vi "Car Wash.vi"() -> ()   [LabVIEW 2020]
uses:
  Controls/Car Wash Indicators.ctl
  Controls/Wash Options.ctl
  Controls/Car Wash References.ctl
  Controls/Wash Steps Selected-Update Display Message.ctl
  Controls/Timer Controls.ctl
  Support/Enqueue Message (Single).vi
  <vilib>/Utility/error.llb/Error Cluster From Error Code.vi
  <vilib>/ErrorRing/Error Ring.xnode
  Support/Message Queue.lvlib
panel:
  in  "Start":bool
  out "Elapsed Time":dbl format="%0.2f"
  in  "stop":bool
  out "Wash Entry":bool
  in  "Wash Options":T1
  in  "Car Position Slider":u8(slide) max=3 scale=0.0..4.0
  out "Car Wash Indicators":T2
  # "Entry Console"
  # "Car Wash Display"
  # "Car Position Simulation"
  # "Pre-Soak\nH-P Wash\nL-P Wax\nSpot Free Rinse"
  # "Underbody Wash\nBug Remover"
  # "Tire Shine\nAir Dry"
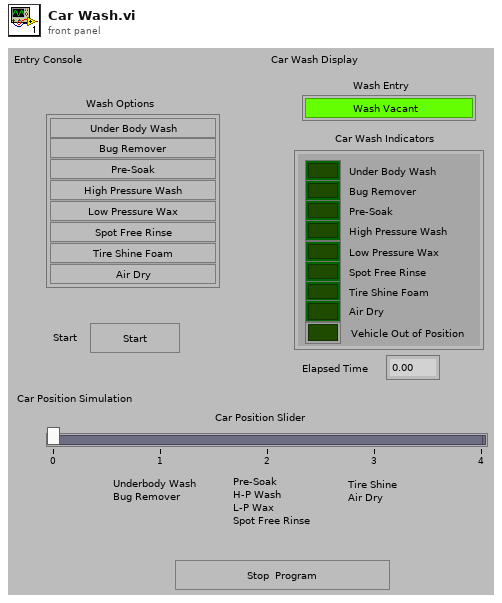
[diagram p1: front panel]
types:
  T1 = typedef "Wash Options.ctl" = cluster{"Underbody Wash":bool, "Bug Remover":bool, "Pre-Soak":bool, "High Pressure Wash":bool, "Low Pressure Wax":bool, "Spot Free Rinse":bool, "Tire Shine Foam":bool, "Air Dry":bool}
  T2 = typedef "Car Wash Indicators.ctl" = cluster{"Under Body Wash":bool, "Bug Remover":bool, "Pre-Soak":bool, "High Pressure Wash":bool, "Low Pressure Wax":bool, "Spot Free Rinse":bool, "Tire Shine Foam":bool, "Air Dry":bool, "Vehicle Out of Position":bool}
  T3 = typedef "Car Wash References.ctl" = cluster{"Car Wash Indicators Ref":refnum<vi>, "Wash Options Ref":refnum<vi>, "Car Position Slider Ref":refnum<vi>, "Elapsed Time Ref":refnum<vi>, "Wash Entry Ref":refnum<vi>, "Start Ref":refnum<vi>}
  T4 = typedef "Message Queue.lvlib/All Message Queues.ctl" = cluster{"UI":refnum<queue>}
  T5 = typedef "Wash Steps Selected-Update Display Message.ctl" = cluster{"Wash Steps Selected":cluster{"Wash Step":string, "Step Time":i32, "Station":string}[], "Update Display Message":string}
  T6 = enum8{"Enabled", "Disabled", "Disabled and Grayed Out"}
  T7 = typedef "Timer Controls.ctl" = enum16{"Reset", "Start", "Stop"}
  T8 = cluster{"Wash Step":string, "Step Time":i32, "Station":string}[]
  T9 = cluster{"Wash Step":string, "Step Time":i32, "Station":string}
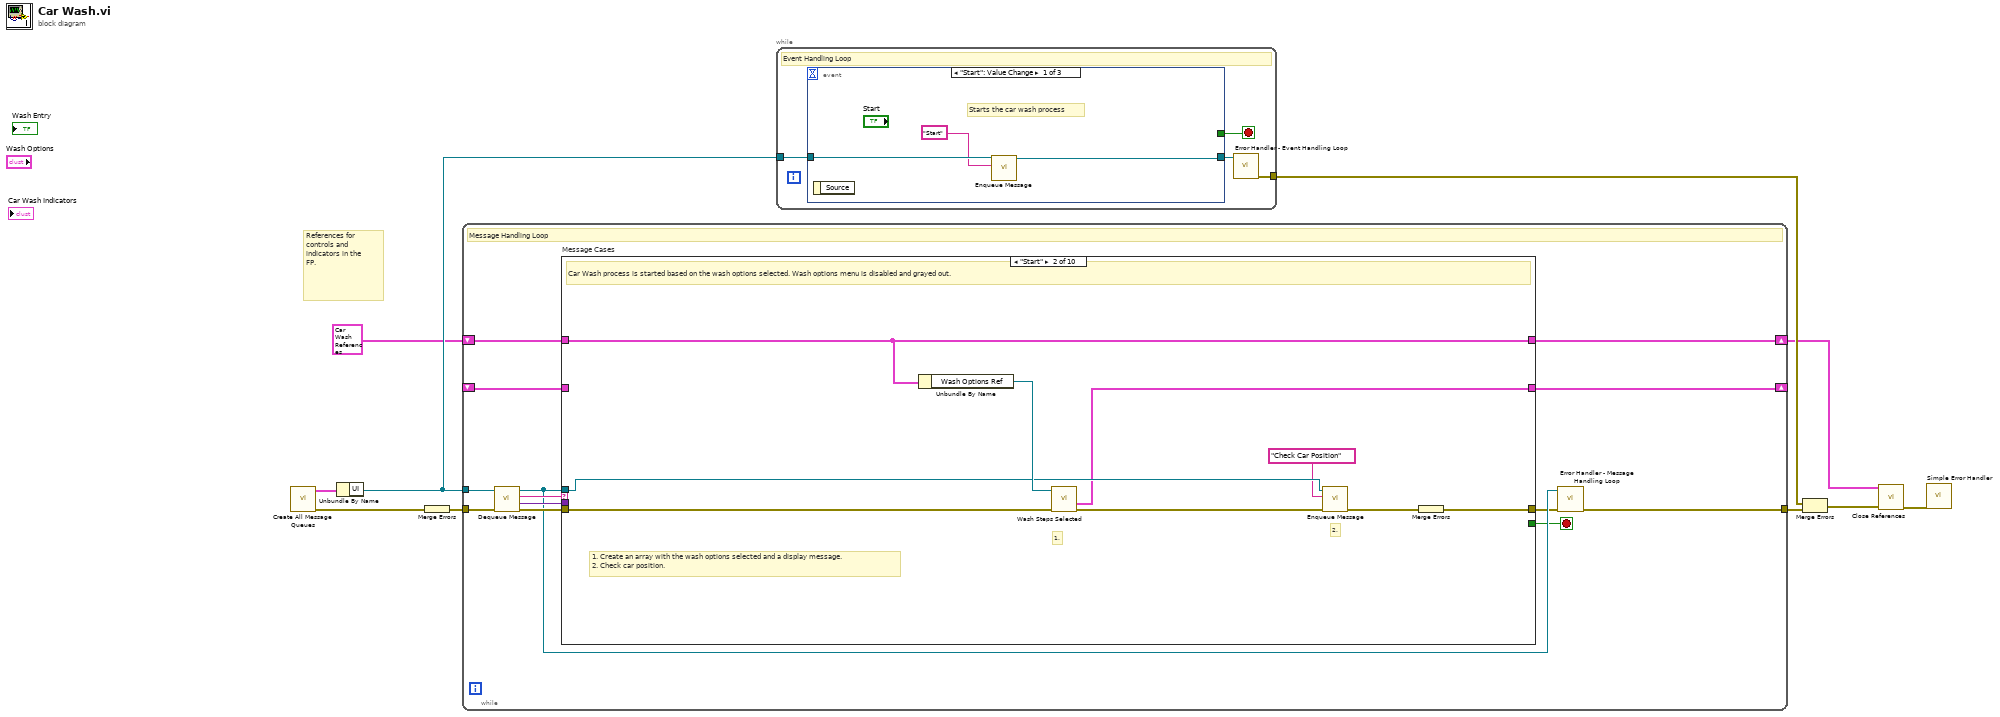
[diagram p0: block diagram]
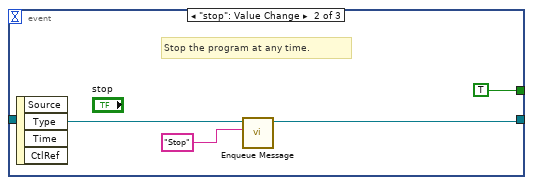
[diagram p2: hidden frame]
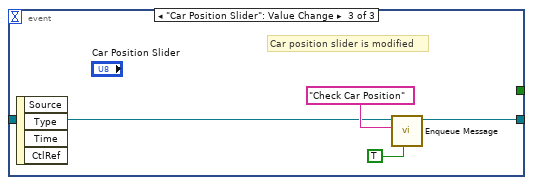
[diagram p3: hidden frame]
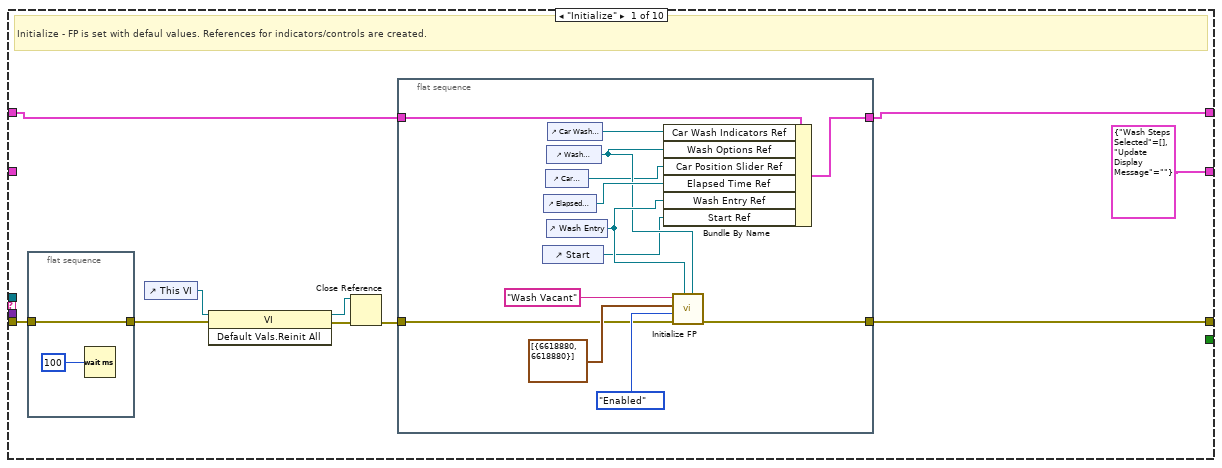
[diagram p4: hidden frame]
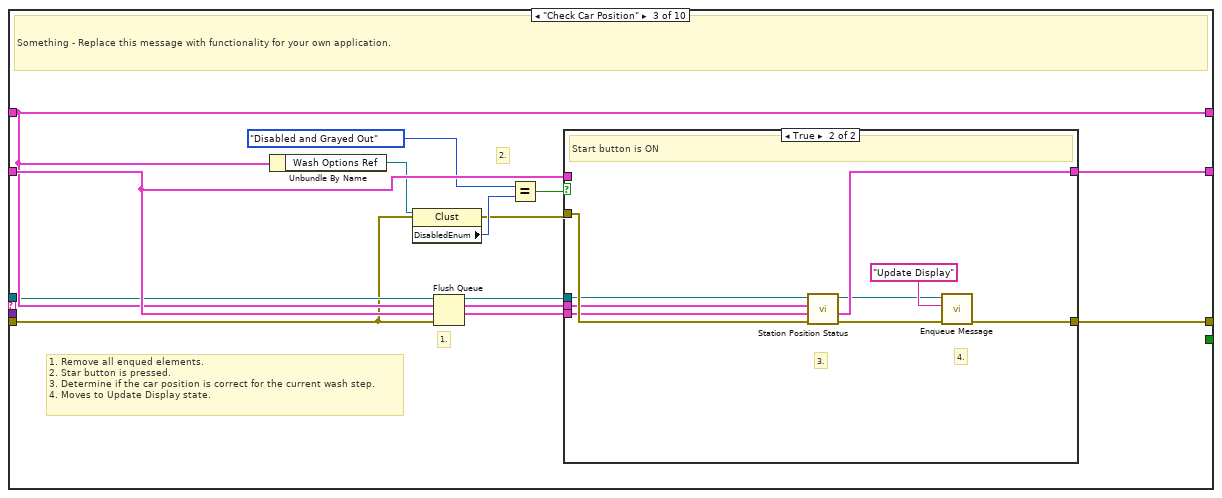
[diagram p5: hidden frame]
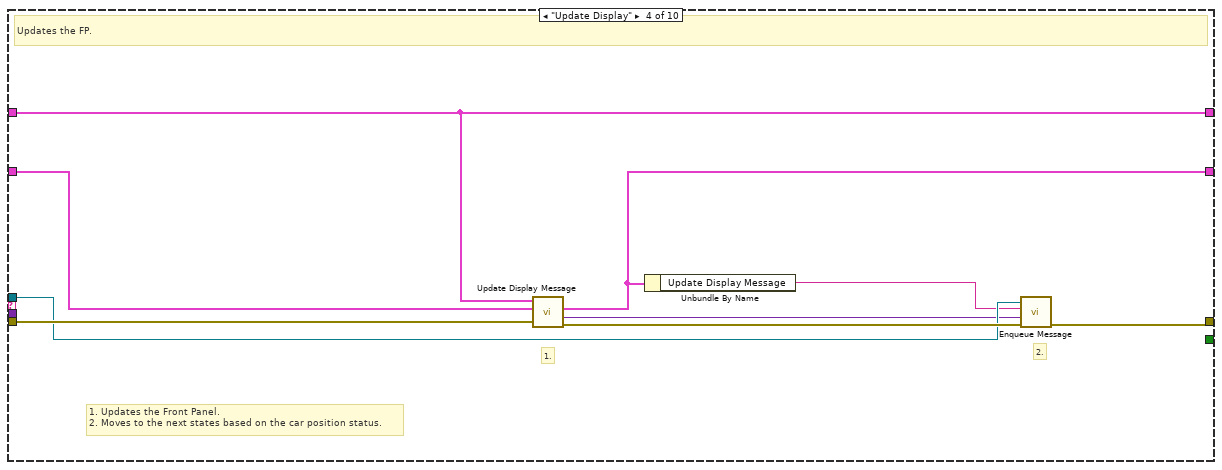
[diagram p7: hidden frame]
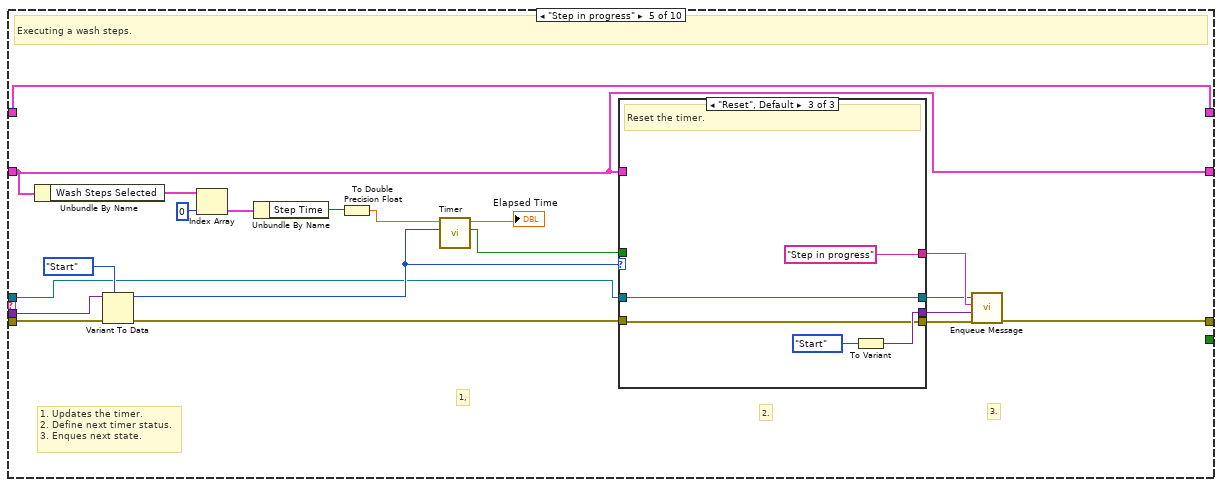
[diagram p8: hidden frame]
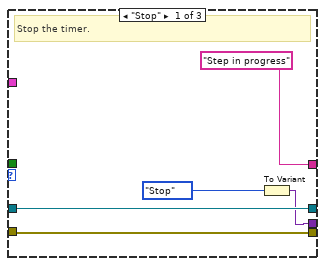
[diagram p9: hidden frame]
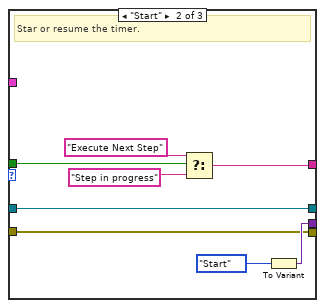
[diagram p10: hidden frame]
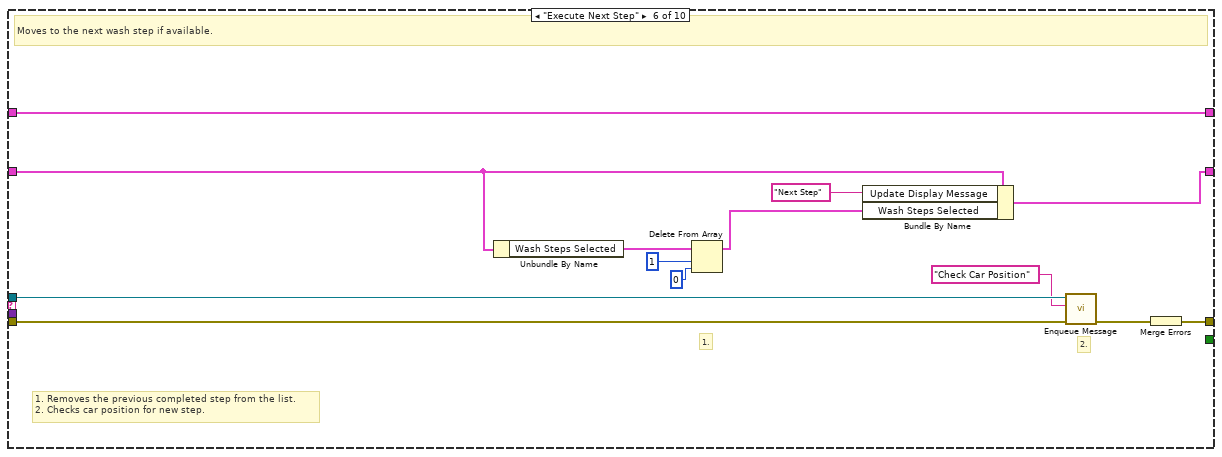
[diagram p11: hidden frame]
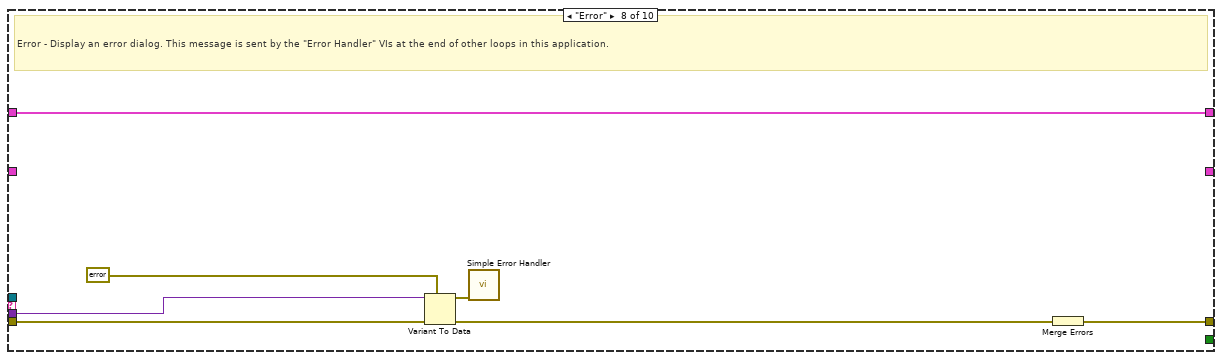
[diagram p13: hidden frame]
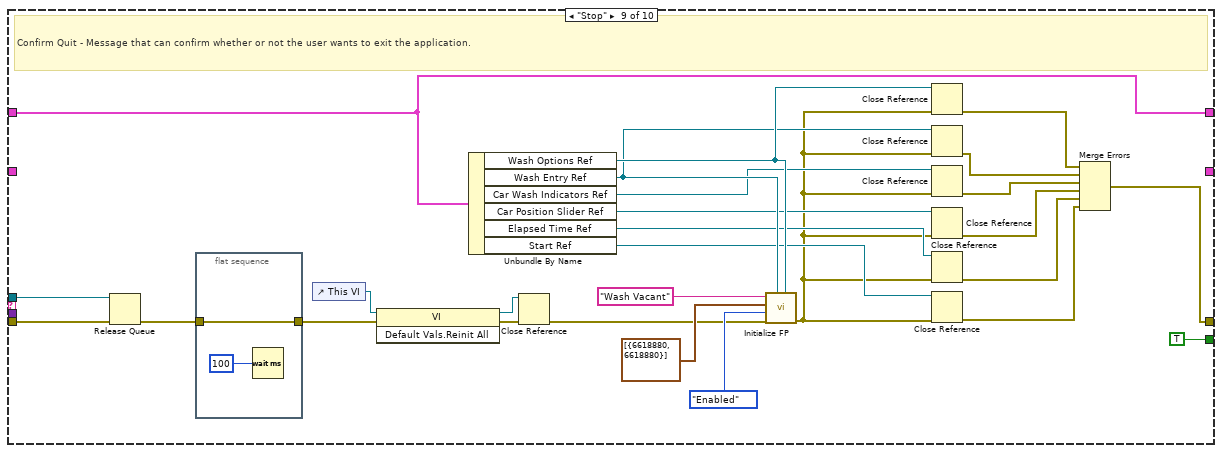
[diagram p14: hidden frame]
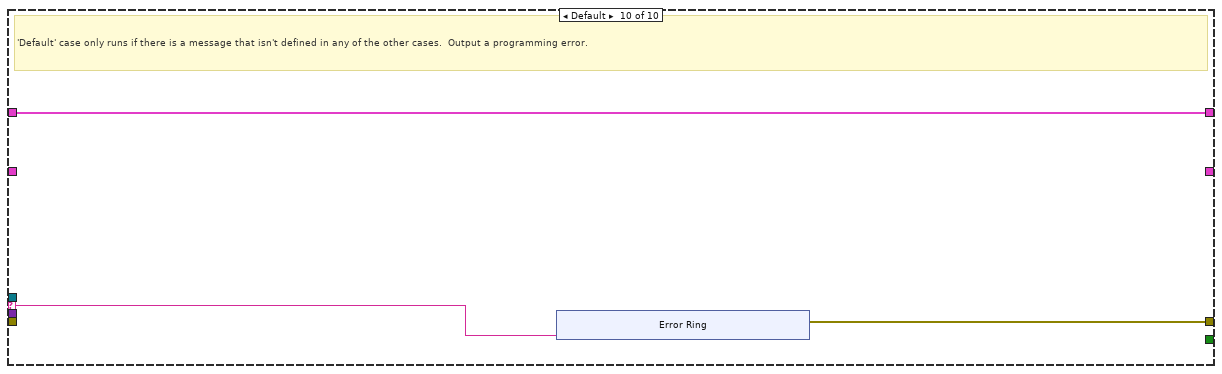
[diagram p15: hidden frame]
diagram:
  # "References for controls and indicators in the FP."
  n1 = call "Create All Message Queues.vi"() -> ("error out"=w10:errorcluster, "Message Queues out"=w9:T4)  [unwired: 10 in]
  n2 = Unbundle By Name(w9) -> ("UI"=w7:refnum<queue>)
  n3 = Merge Errors(w10) -> (w5:errorcluster)
  n4 = while {
    tunnel: w7 -> [w17]
    shift-right: [w22] -> w3
    shift-left: T3 {"Car Wash Indicators Ref"=refnum, "Wash Options Ref"=refnum, "Car Position Slider Ref"=refnum, "Elapsed Time Ref"=refnum, "Wash Entry Ref"=refnum, "Start Ref"=refnum} ("Data Cluster") -> [w23]
    tunnel: w5 -> [w21]
    tunnel: [w15] -> w8
    shift-right: [w12] -> _
    shift-left: _ -> [w11]
    stop <- w13 stop-if-true
    # "Message Handling Loop"
    n5 = call "Dequeue Message.vi"("error in (no error)"=w21, "Message Queue"=w17) -> ("error out"=w20:errorcluster, "Message Data"=w18:variant, "Message"=w19:string, "dup Message Queue"=w16:refnum<queue>)  [unwired: 6 in]
    n6 = case "Message Cases" shown="\"Start\"" w19 {
      selector: w19 -> [_ _ _ _ _ _ _ _ _ w179]
      tunnel: w16 -> [_ w52 w59 w84 w93 w136 _ _ w175 _]
      tunnel: w20 -> [w28 w55 w58 w88 w102 w128 w140 w149 w174 _]
      tunnel: [w29 w57 w69 w85 w94 w138 w140 w143 w151 w180] -> w14
      tunnel: w23 -> [w33 w56 w66 w87 w108 w139 w142 w148 w150 w181]
      tunnel: [w31 w56 w66 w87 w108 w139 w142 w148 w150 w181] -> w22
      tunnel: w18 -> [_ _ _ _ w103 _ _ w147 _ _]
      tunnel: [_ _ _ _ _ _ _ _ TRUE _] -> w13
      tunnel: [T5 {"Wash Steps Selected"=[], "Update Display Message"=""} ("Wash Steps Selected-Update Display Message") w50 w68 w81 w91 w127 w141 _ _ _] -> w12
      tunnel: w11 -> [_ _ w67 w82 w91 w131 w141 _ _ _]
      frame "Initialize" {
        # "Initialize - FP is set with defaul values. References for indicators/controls are created."
        n7 = flat-sequence {
          tunnel: w28 -> [w34]
          tunnel: [w34] -> w27
          frame #0 {
            n8 = Wait (ms)(milliseconds to wait=u32 100) -> ()  [unwired: 1 out]
          }
        }
        n9 = control-ref of="This VI"() -> (w30:refnum<vi>)
        n10 = invoke class="VI" method="Default Vals.Reinit All"(reference=w30, error in=w27) -> (reference out=w24:refnum<vi>, error out=w25:errorcluster)  [unwired: 1 in, 1 out]
        n11 = Close Reference(reference=w24, error in (no error)=w25) -> (error out=w26:errorcluster)
        n12 = flat-sequence {
          tunnel: w33 -> [w48]
          tunnel: [w39] -> w31
          tunnel: w26 -> [w38]
          tunnel: [w37] -> w29
          frame #0 {
            n13 = control-ref of="Start"() -> (w41:refnum<vi>)
            n14 = control-ref of="Elapsed Time"() -> (w47:refnum<vi>)
            n15 = control-ref of="Car Position Slider"() -> (w36:refnum<vi>)
            n16 = control-ref of="Wash Options"() -> (w42:refnum<vi>)
            n17 = control-ref of="Wash Entry"() -> (w43:refnum<vi>)
            n18 = control-ref of="Car Wash Indicators"() -> (w46:refnum<vi>)
            n19 = Bundle By Name(cluster=w48, "Car Wash Indicators Ref"=w46, "Wash Options Ref"=w42, "Car Position Slider Ref"=w36, "Elapsed Time Ref"=w47, "Wash Entry Ref"=w43, "Start Ref"=w41) -> (w39:T3)
            n20 = call "Initialize FP.vi"("Wash Options Ref"=w42, "Wash Entry Ref"=w43, "error in"=w38, "Enable\\Disable Wash Options"=T6."Enabled" ("Enable\\Disable Wash Options"), "Wash In Progress Color"=cluster{u32, u32}[] [{6618880, 6618880}], "Wash In Progress Text"="Wash Vacant") -> ("error out"=w37:errorcluster)  [unwired: 5 in]
          }
        }
      }
      frame "Start" {
        # "1. Create an array with the wash options selected and a display message.\n2. Check car position."
        # "2."
        # "1."
        # "Car Wash process is started based on the wash options selected. Wash options menu is disabled and grayed out."
        n21 = Unbundle By Name(w56) -> ("Wash Options Ref"=w54:refnum<vi>)
        n22 = call "Wash Steps Selected.vi"("error in (no error)"=w55, "Wash Options Ref"=w54) -> ("error out"=w49:errorcluster, "Wash Steps Selected-Update Display Message"=w50:T5)  [unwired: 8 in]
        n23 = call-poly "Enqueue Message.vi"("error in (no error)"=w49, "Message"="Check Car Position", "Message Queue"=w52) -> ("error out"=w53:errorcluster)  [unwired: 7 in, 1 out]
        n24 = Merge Errors(w53) -> (w57:errorcluster)
      }
      frame "Check Car Position" {
        # "1. Remove all enqued elements.\n2. Star button is pressed.\n3. Determine if the car position is correct for the current wash step. \n4. Moves to Update Display state."
        # "1."
        # "2."
        # "Something - Replace this message with functionality for your own application."
        n25 = Unbundle By Name(w66) -> ("Wash Options Ref"=w65:refnum<vi>)
        n26 = property class="Clust"(reference=w65, error in=w58) -> (error out=w61:errorcluster, "DisabledEnum"=w63:T6)  [unwired: 1 out]
        n27 = Flush Queue(queue=w59, error in (no error)=w58) -> (queue out=w60:refnum<queue>)  [unwired: 2 out]
        n28 = Equal?(x=T6."Disabled and Grayed Out", y=w63) -> (x = y?=w64:bool)
        n29 = case shown="True" w64 {
          tunnel: [w70 w76] -> w69
          tunnel: w60 -> [_ w72]
          tunnel: w66 -> [_ w73]
          tunnel: w67 -> [_ w74]
          tunnel: [w71 w77] -> w68
          tunnel: w67 -> [w71 _]
          tunnel: w61 -> [w70 w75]
          frame False {
            # "Start button is OFF"
          }
          frame True {
            # "4."
            # "3."
            # "Start button is ON"
            n30 = call "Station Position Status.vi"("error in (no error)"=w75, "Wash Steps Selected-Update Display Message"=w74, "Car Wash References"=w73) -> ("error out"=w79:errorcluster, "Message Out"=w77:T5)  [unwired: 5 in]
            n31 = call-poly "Enqueue Message.vi"("error in (no error)"=w79, "Message"="Update Display", "Message Queue"=w72) -> ("error out"=w76:errorcluster)  [unwired: 7 in, 1 out]
          }
        }
      }
      frame "Update Display" {
        # "1. Updates the Front Panel.\n2. Moves to the next states based on the car position status."
        # "2."
        # "1."
        # "Updates the FP."
        n32 = call "Update Display Message.vi"("error in (no error)"=w88, "Wash Steps Selected-Update Display Message In"=w82, "Data Cluster"=w87) -> ("error out"=w86:errorcluster, "Step in progress timer control"=w80:variant, "Wash Steps Selected-Update Display Message Out"=w81:T5)  [unwired: 6 in]
        n33 = Unbundle By Name(w81) -> ("Update Display Message"=w83:string)
        n34 = call-poly "Enqueue Message.vi"("error in (no error)"=w86, "Message Data"=w80, "Message"=w83, "Message Queue"=w84) -> ("error out"=w85:errorcluster)  [unwired: 6 in, 1 out]
      }
      frame "Step in progress" {
        # "1. Updates the timer.\n2. Define next timer status.\n3. Enques next state."
        # "3."
        # "2."
        # "1,"
        # "Executing a wash steps."
        n35 = Unbundle By Name(w91) -> ("Wash Steps Selected"=w107:T8)
        n36 = Variant To Data(error in=w102, type=Timer_Controls."Start", Variant=w103) -> (data=w100:T7, error out=w101:errorcluster)
        n37 = Index Array(array=w107, index=0) -> (element=w105:T9)
        n38 = Unbundle By Name(w105) -> ("Step Time"=w104:i32)
        n39 = To Double Precision Float(number=w104) -> (double precision float=w90:dbl)
        n40 = call "Timer.vi"("Timer Control"=w100, "Time Target"=w90) -> ("Time completed?"=w99:bool, "Elapsed Time"=→"Elapsed Time":dbl)  [unwired: 8 in]
        n41 = case shown="\"Reset\", Default" w100 {
          tunnel: w93 -> [w112 w116 w125]
          tunnel: w101 -> [w113 w117 w123]
          tunnel: [w113 w117 w123] -> w89
          tunnel: w99 -> [_ w119 _]
          tunnel: [w110 w118 w124] -> w96
          tunnel: ["Step in progress" ("Message") w115 "Step in progress" ("Message")] -> w95
          tunnel: [w112 w116 w125] -> w92
          tunnel: w91 -> [_ _ _]
          frame "Stop" {
            # "Stop the timer."
            n42 = To Variant(anything=Timer_Controls."Stop" ("Enum")) -> (Variant=w110:variant)
          }
          frame "Start" {
            # "Star or resume the timer."
            n43 = Select(t="Execute Next Step" ("Message"), s=w119, f="Step in progress" ("Message")) -> (s? t:f=w115:string)
            n44 = To Variant(anything=Timer_Controls."Start" ("Enum")) -> (Variant=w118:variant)
          }
          frame "Reset", Default {
            # "Reset the timer."
            n45 = To Variant(anything=Timer_Controls."Start" ("Enum")) -> (Variant=w124:variant)
          }
        }
        n46 = call-poly "Enqueue Message.vi"("error in (no error)"=w89, "Message Data"=w96, "Message"=w95, "Message Queue"=w92) -> ("error out"=w94:errorcluster)  [unwired: 6 in, 1 out]
      }
      frame "Execute Next Step" {
        # "1. Removes the previous completed step from the list.\n2. Checks car position for new step."
        # "2."
        # "1."
        # "Moves to the next wash step if available."
        n47 = Unbundle By Name(w131) -> ("Wash Steps Selected"=w129:T8)
        n48 = Delete From Array(array=w129, length=1, index=0) -> (array with subset deleted=w130:T8)  [unwired: 1 out]
        n49 = Bundle By Name(cluster=w131, "Update Display Message"="Next Step", "Wash Steps Selected"=w130) -> (w127:T5)
        n50 = call-poly "Enqueue Message.vi"("error in (no error)"=w128, "Message"="Check Car Position", "Message Queue"=w136) -> ("error out"=w137:errorcluster)  [unwired: 7 in, 1 out]
        n51 = Merge Errors(w137) -> (w138:errorcluster)
      }
      frame "Vehicle Out of Position" {
        # "Vehicle is Out of Position. Waiting for the right Car position."
      }
      frame "Error" {
        # "Error - Display an error dialog. This message is sent by the \"Error Handler\" VIs at the end of other loops in this application."
        n52 = Variant To Data(error in=w149, type=errorcluster {"status"=FALSE, "code"=0, "source"=""} ("error constant"), Variant=w147) -> (data=w145:errorcluster, error out=w144:errorcluster)
        n53 = call <vilib>:"Simple Error Handler.vi"("error in (no error)"=w145) -> ()  [unwired: 4 in, 5 out]
        n54 = Merge Errors(w144) -> (w143:errorcluster)
      }
      frame "Stop" {
        # "Confirm Quit - Message that can confirm whether or not the user wants to exit the application."
        n55 = Release Queue(queue=w175, error in (no error)=w174) -> (error out=w170:errorcluster)  [unwired: 1 in, 2 out]
        n56 = flat-sequence {
          tunnel: w170 -> [w177]
          tunnel: [w177] -> w169
          frame #0 {
            n57 = Wait (ms)(milliseconds to wait=u32 100) -> ()  [unwired: 1 out]
          }
        }
        n58 = control-ref of="This VI"() -> (w173:refnum<vi>)
        n59 = invoke class="VI" method="Default Vals.Reinit All"(reference=w173, error in=w169) -> (reference out=w171:refnum<vi>, error out=w172:errorcluster)  [unwired: 1 in, 1 out]
        n60 = Unbundle By Name(w150) -> ("Wash Options Ref"=w164:refnum<vi>, "Wash Entry Ref"=w163:refnum<vi>, "Car Wash Indicators Ref"=w162:refnum<vi>, "Car Position Slider Ref"=w161:refnum<vi>, "Elapsed Time Ref"=w160:refnum<vi>, "Start Ref"=w159:refnum<vi>)
        n61 = Close Reference(reference=w171, error in (no error)=w172) -> (error out=w165:errorcluster)
        n62 = call "Initialize FP.vi"("Wash Options Ref"=w164, "Wash Entry Ref"=w163, "error in"=w165, "Enable\\Disable Wash Options"=T6."Enabled" ("Enable\\Disable Wash Options"), "Wash In Progress Color"=cluster{u32, u32}[] [{6618880, 6618880}], "Wash In Progress Text"="Wash Vacant") -> ("error out"=w158:errorcluster)  [unwired: 5 in]
        n63 = Close Reference(reference=w164, error in (no error)=w158) -> (error out=w157:errorcluster)
        n64 = Close Reference(reference=w163, error in (no error)=w158) -> (error out=w156:errorcluster)
        n65 = Close Reference(reference=w162, error in (no error)=w158) -> (error out=w155:errorcluster)
        n66 = Close Reference(reference=w161, error in (no error)=w158) -> (error out=w154:errorcluster)
        n67 = Close Reference(reference=w160, error in (no error)=w158) -> (error out=w153:errorcluster)
        n68 = Close Reference(reference=w159, error in (no error)=w158) -> (error out=w152:errorcluster)
        n69 = Merge Errors(w157, w156, w155, w154, w153, w152) -> (w151:errorcluster)
      }
      frame Default {
        # "'Default' case only runs if there is a message that isn't defined in any of the other cases.  Output a programming error."
        n70 = xnode "Error Ring"("parameter 0"=w179) -> ("error out"=w180:errorcluster)
      }
    }
    n71 = call "Error Handler - Message Handling Loop.vi"("error in (no error)"=w14, "Message Queue"=w16) -> ("dup error in"=w15:errorcluster)  [unwired: 8 in, 1 out]
  }
  n72 = while {
    tunnel: w7 -> [w192]
    tunnel: [w189] -> w4
    stop <- w191 stop-if-true
    # "Event Handling Loop"
    n73 = event shown="[0] \"Start\": Value Change" {
      selector: _ -> [_ _ _]
      dyn-events: _ -> [_ _ _]
      timeout: _ -> [_ _ _]
      tunnel: [_ TRUE ("Discard?") _] -> w191
      tunnel: w192 -> [w195 w198 w201]
      tunnel: [w194 w197 w203] -> w190
      event "Start": Value Change {
        # "Starts the car wash process"
        n74 = event-data() -> ()  [unwired: 1 in, 1 out]
        n75 = call-poly "Enqueue Message.vi"("Message"="Start", "Message Queue"=w195) -> ("dup Message Queue"=w194:refnum<queue>)  [unwired: 8 in, 1 out]
      }
      event "stop": Value Change {
        # "Stop the program at any time."
        n76 = event-data() -> ()  [unwired: 1 in, 4 out]
        n77 = call-poly "Enqueue Message.vi"("Message"="Stop", "Message Queue"=w198) -> ("dup Message Queue"=w197:refnum<queue>)  [unwired: 8 in, 1 out]
      }
      event "Car Position Slider": Value Change {
        # "Car position slider is modified"
        n78 = event-data() -> ()  [unwired: 1 in, 4 out]
        n79 = call-poly "Enqueue Message.vi"("Priority Message? (F)"=TRUE, "Message"="Check Car Position", "Message Queue"=w201) -> ("dup Message Queue"=w203:refnum<queue>)  [unwired: 7 in, 1 out]
      }
    }
    n80 = call "Error Handler - Event Handling Loop.vi"("Message Queue"=w190) -> ("dup error in"=w189:errorcluster)  [unwired: 9 in, 1 out]
  }
  n81 = Merge Errors(w4, w8) -> (w2:errorcluster)
  n82 = call "Close References.vi"("error in"=w2, "References"=w3) -> ("error out"=w1:errorcluster)  [unwired: 9 in]
  n83 = call <vilib>:"Simple Error Handler.vi"("error in (no error)"=w1) -> ()  [unwired: 4 in, 5 out]
